vi "Bass Subvi3.vi"(0 "Image Dst Out":T2) -> (9 "Orange Bass LED":bool, 11 "Red Bass LED":bool, 13 "Green Bass LED":bool, 15 "Yellow Bass LED":bool, 19 "Blue Bass LED":bool)   [LabVIEW 2009]
uses:
  <vilib>/vision/Image Controls.llb/IMAQ Image.ctl
  <vilib>/Analysis/3filter.llb/Filter Passband Type.ctl
  <vilib>/Analysis/3filter.llb/Butterworth Filter (DBL).vi
  <vilib>/Analysis/NI_AALBase.lvlib
  <vilib>/vision/NI_Vision_Development_Module.lvlib
panel:
  in  "Blue Bass 2":T1={"Global Rectangle"=[192, 292, 199, 386], "Contours"=[{"ID"=enum."External", "Type"=2, "Coordinates"=[192, 385, 198, 292]}]} {"Contours"."Type" items=["No Selection", "Point", "Line", "Rectangle", "Oval", "Polygon", "Freehand Region", "Annulus", "Unused2", "Unused3", "Broken Line", "Freehand Line", "Rotated Rectangle"]}
  in  "Orange Bass 2":T1={"Global Rectangle"=[220, 302, 227, 392], "Contours"=[{"ID"=enum."External", "Type"=2, "Coordinates"=[226, 391, 220, 302]}]} {"Contours"."Type" items=["No Selection", "Point", "Line", "Rectangle", "Oval", "Polygon", "Freehand Region", "Annulus", "Unused2", "Unused3", "Broken Line", "Freehand Line", "Rotated Rectangle"]}
  in  "Green Bass 2":T1={"Global Rectangle"=[100, 292, 131, 371], "Contours"=[{"ID"=enum."External", "Type"=2, "Coordinates"=[100, 370, 130, 292]}]} {"Contours"."Type" items=["No Selection", "Point", "Line", "Rectangle", "Oval", "Polygon", "Freehand Region", "Annulus", "Unused2", "Unused3", "Broken Line", "Freehand Line", "Rotated Rectangle"]}
  in  "Red Bass 2":T1={"Global Rectangle"=[129, 294, 154, 376], "Contours"=[{"ID"=enum."External", "Type"=2, "Coordinates"=[129, 375, 153, 294]}]} {"Contours"."Type" items=["No Selection", "Point", "Line", "Rectangle", "Oval", "Polygon", "Freehand Region", "Annulus", "Unused2", "Unused3", "Broken Line", "Freehand Line", "Rotated Rectangle"]}
  in  "Yellow Bass 2":T1={"Global Rectangle"=[160, 295, 175, 378], "Contours"=[{"ID"=enum."External", "Type"=2, "Coordinates"=[160, 377, 174, 295]}]} {"Contours"."Type" items=["No Selection", "Point", "Line", "Rectangle", "Oval", "Polygon", "Freehand Region", "Annulus", "Unused2", "Unused3", "Broken Line", "Freehand Line", "Rotated Rectangle"]}
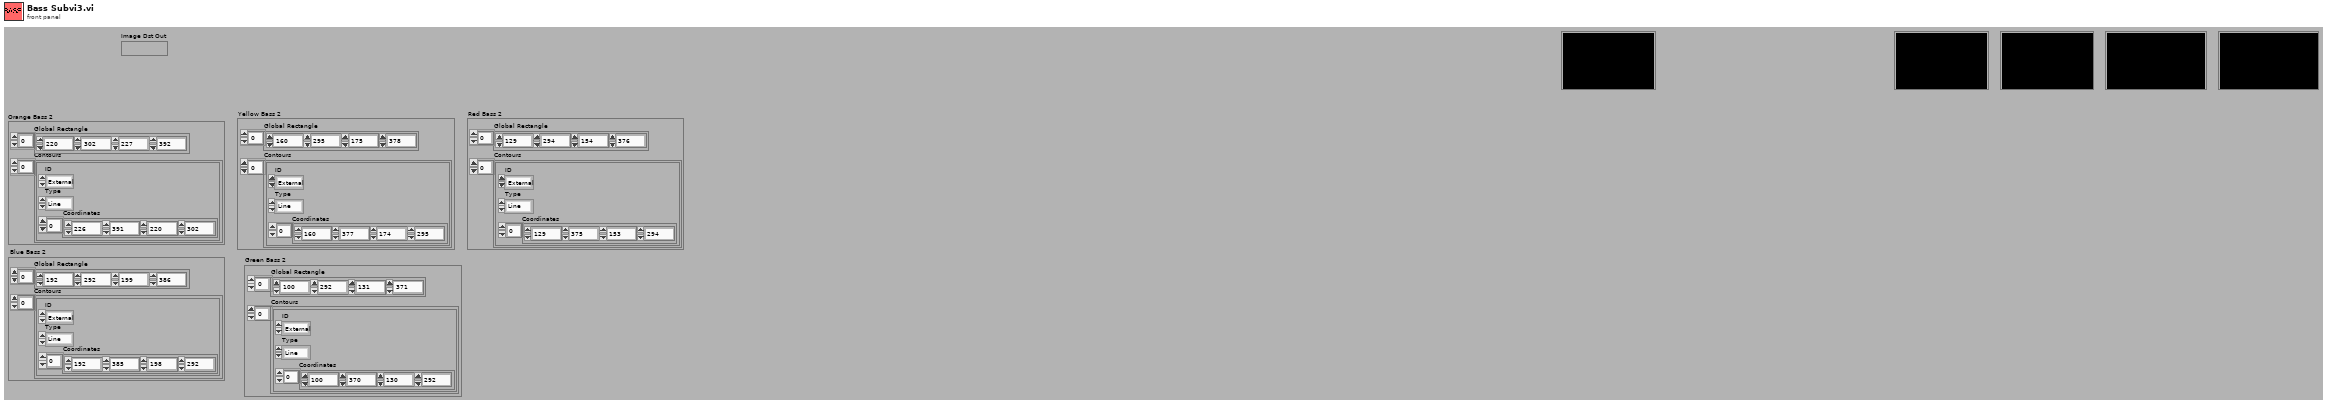
[diagram p1: front panel]
types:
  T1 = cluster{"Global Rectangle":i32[], "Contours":cluster{"ID":enum32{"External", "Internal"}, "Type":u32, "Coordinates":i32[]}[]}
  T2 = typedef "IMAQ Image.ctl" = refnum<image>
  T3 = typedef "NI_AALBase.lvlib/Filter Passband Type.ctl" = enum32{"Lowpass", "Highpass", "Bandpass", "Bandstop"}
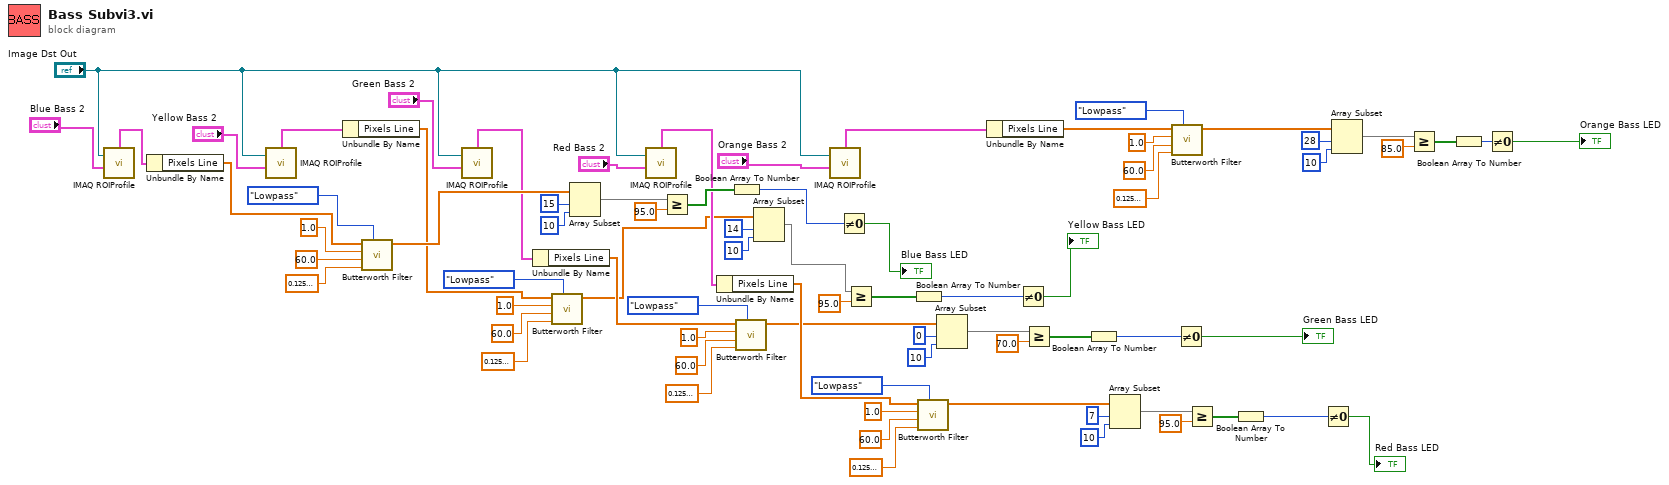
[diagram p0: block diagram]
diagram:
  n1 = call "IMAQ ROIProfile"("ROI Descriptor"="Blue Bass 2", "Image"="Image Dst Out") -> ("ROI Graph"=w27:cluster{"x0":sgl, "dx":sgl, "Pixels Line":sgl[]})  [unwired: 1 in, 5 out]
  n2 = Unbundle By Name(w27) -> ("Pixels Line"=w6:sgl[])
  n3 = call "IMAQ ROIProfile"("ROI Descriptor"="Yellow Bass 2", "Image"="Image Dst Out") -> ("ROI Graph"=w24:cluster{"x0":sgl, "dx":sgl, "Pixels Line":sgl[]})  [unwired: 1 in, 5 out]
  n4 = Unbundle By Name(w24) -> ("Pixels Line"=w21:sgl[])
  n5 = call-poly <vilib>:"Butterworth Filter.vi"("filter type"=Filter_Passband_Type."Lowpass", "low cutoff freq: fl"=0.12500000000000006 ("low 2"), "high cutoff freq: fh"=60.0 ("high 8"), "sampling freq: fs"=1.0 ("sampling  8"), "X"=w6) -> ("Filtered X"=w41:dbl[])  [unwired: 3 in, 1 out]
  n6 = call "IMAQ ROIProfile"("ROI Descriptor"="Green Bass 2", "Image"="Image Dst Out") -> ("ROI Graph"=w29:cluster{"x0":sgl, "dx":sgl, "Pixels Line":sgl[]})  [unwired: 1 in, 5 out]
  n7 = Unbundle By Name(w29) -> ("Pixels Line"=w32:sgl[])
  n8 = call-poly <vilib>:"Butterworth Filter.vi"("filter type"=Filter_Passband_Type."Lowpass", "low cutoff freq: fl"=0.12500000000000006 ("low  7"), "high cutoff freq: fh"=60.0 ("high 7"), "sampling freq: fs"=1.0 ("sampling 7"), "X"=w21) -> ("Filtered X"=w25:dbl[])  [unwired: 3 in, 1 out]
  n9 = Array Subset(array=w41, index=15, length=10) -> (w12:dbl[])
  n10 = call "IMAQ ROIProfile"("ROI Descriptor"="Red Bass 2", "Image"="Image Dst Out") -> ("ROI Graph"=w53:cluster{"x0":sgl, "dx":sgl, "Pixels Line":sgl[]})  [unwired: 1 in, 5 out]
  n11 = Greater Or Equal?(x=w12, y=95.0) -> (x >= y?=w75:bool[])
  n12 = Unbundle By Name(w53) -> ("Pixels Line"=w50:sgl[])
  n13 = Boolean Array To Number(Boolean array=w75) -> (number=w14:u32)
  n14 = call-poly <vilib>:"Butterworth Filter.vi"("filter type"=Filter_Passband_Type."Lowpass", "low cutoff freq: fl"=0.12500000000000006 ("low  6"), "high cutoff freq: fh"=60.0 ("high 6"), "sampling freq: fs"=1.0 ("sampling 6"), "X"=w32) -> ("Filtered X"=w28:dbl[])  [unwired: 3 in, 1 out]
  n15 = Array Subset(array=w25, index=14, length=10) -> (w1:dbl[])
  n16 = call "IMAQ ROIProfile"("ROI Descriptor"="Orange Bass 2", "Image"="Image Dst Out") -> ("ROI Graph"=w59:cluster{"x0":sgl, "dx":sgl, "Pixels Line":sgl[]})  [unwired: 1 in, 5 out]
  n17 = Not Equal To 0?(x=w14) -> (x != 0?=→"Blue Bass LED":bool)
  n18 = Greater Or Equal?(x=w1, y=95.0) -> (x >= y?=w18:bool[])
  n19 = Boolean Array To Number(Boolean array=w18) -> (number=w19:u32)
  n20 = call-poly <vilib>:"Butterworth Filter.vi"("filter type"=Filter_Passband_Type."Lowpass", "low cutoff freq: fl"=0.12500000000000006 ("low  5"), "high cutoff freq: fh"=60.0 ("high 5"), "sampling freq: fs"=1.0 ("sampling 5"), "X"=w50) -> ("Filtered X"=w54:dbl[])  [unwired: 3 in, 1 out]
  n21 = Array Subset(array=w28, index=0, length=10) -> (w37:dbl[])
  n22 = Unbundle By Name(w59) -> ("Pixels Line"=w62:sgl[])
  n23 = Not Equal To 0?(x=w19) -> (x != 0?=→"Yellow Bass LED":bool)
  n24 = Greater Or Equal?(x=w37, y=70.0) -> (x >= y?=w35:bool[])
  n25 = Boolean Array To Number(Boolean array=w35) -> (number=w34:u32)
  n26 = Array Subset(array=w54, index=7, length=10) -> (w45:dbl[])
  n27 = call-poly <vilib>:"Butterworth Filter.vi"("filter type"=Filter_Passband_Type."Lowpass", "low cutoff freq: fl"=0.12500000000000006 ("low  8"), "high cutoff freq: fh"=60.0 ("high 9"), "sampling freq: fs"=1.0 ("sampling 8"), "X"=w62) -> ("Filtered X"=w58:dbl[])  [unwired: 3 in, 1 out]
  n28 = Not Equal To 0?(x=w34) -> (x != 0?=→"Green Bass LED":bool)
  n29 = Greater Or Equal?(x=w45, y=95.0) -> (x >= y?=w47:bool[])
  n30 = Boolean Array To Number(Boolean array=w47) -> (number=w48:u32)
  n31 = Not Equal To 0?(x=w48) -> (x != 0?=→"Red Bass LED":bool)
  n32 = Array Subset(array=w58, index=28, length=10) -> (w67:dbl[])
  n33 = Greater Or Equal?(x=w67, y=85.0) -> (x >= y?=w65:bool[])
  n34 = Boolean Array To Number(Boolean array=w65) -> (number=w64:u32)
  n35 = Not Equal To 0?(x=w64) -> (x != 0?=→"Orange Bass LED":bool)
